vi "Configure DUT Thermal Constant.vi"(8 "error in (no error)":errorcluster, 9 "DUT Thermal Constant (100)":i16=100 min=20 max=500, 11 "VISA resource name":refnum<visa-resource-name>) -> (0 "error out":errorcluster, 3 "VISA resource name out":refnum<visa-resource-name>)   [LabVIEW 2012, in "Temptronic TP04300.lvlib"]
doc: "This VI configures DUT thermal constant of TP04300 instrument.\n\n<b>DUT Thermal Constant</b> configures the DUT Thermal constant.\n\nDefault Value: 100 \nValid Range: 20 - 500"
uses:
  <instrlib>/Temptronic TP04300/Temptronic TP04300.lvlib
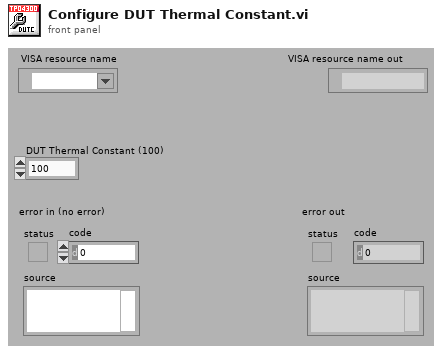
[diagram p1: front panel]
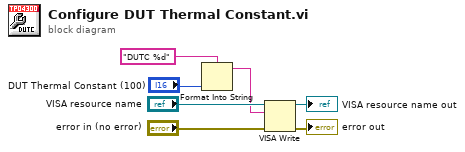
[diagram p0: block diagram]
diagram:
  n1 = Format Into String(format string="DUTC %d" ("multi-line string"), "DUT Thermal Constant (100)") -> (resulting string=w3:string)  [unwired: 2 in, 1 out]
  n2 = VISA Write(VISA resource name="VISA resource name", write buffer=w3, error in (no error)="error in (no error)") -> (VISA resource name out=→"VISA resource name out":refnum<visa-resource-name>, error out=→"error out":errorcluster)  [unwired: 1 out]
